vi "GV-MouseUP.vi"(7 "MouseLeave?":bool, 8 "error in (no error)":errorcluster, 9 "Coords":T1, 11 "Gviewer in":refnum<class "Gviewer.lvclass">) -> (0 "error out":errorcluster, 3 "Gviewer out":refnum<class "Gviewer.lvclass">)   [LabVIEW 2020, in "Sgraph_lib_V1.lvlib" / "Gviewer.lvclass"]
doc: "Andre Koelewijn, 24 jan 2021\n\nAction when in the Gviewer graph the mouse button is released"
uses:
  Gviewer.lvclass
  <vilib>/Utility/miscctls.llb/LVPoint32TypeDef.ctl
  Gviewer.lvclass/Gviewer.ctl
  <vilib>/Utility/cursorutil.llb/Set Cursor (Icon Pict).vi
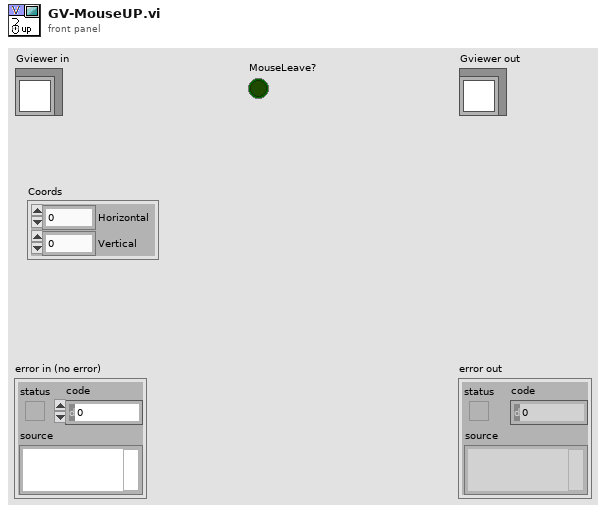
[diagram p1: front panel]
types:
  T1 = typedef "LVPoint32TypeDef.ctl" = cluster{"Horizontal":i32, "Vertical":i32}
  T2 = typedef "Sgraph_lib_V1.lvlib/Gviewer.lvclass/Typedef_Live.ctl" = enum16{"Live View", "Freeze"}
  T3 = typedef "LVPositionTypeDef.ctl" = cluster{"Left":i32, "Top":i32}
  T4 = typedef "LVBoundsTypeDef.ctl" = cluster{"Width":u32, "Height":u32}
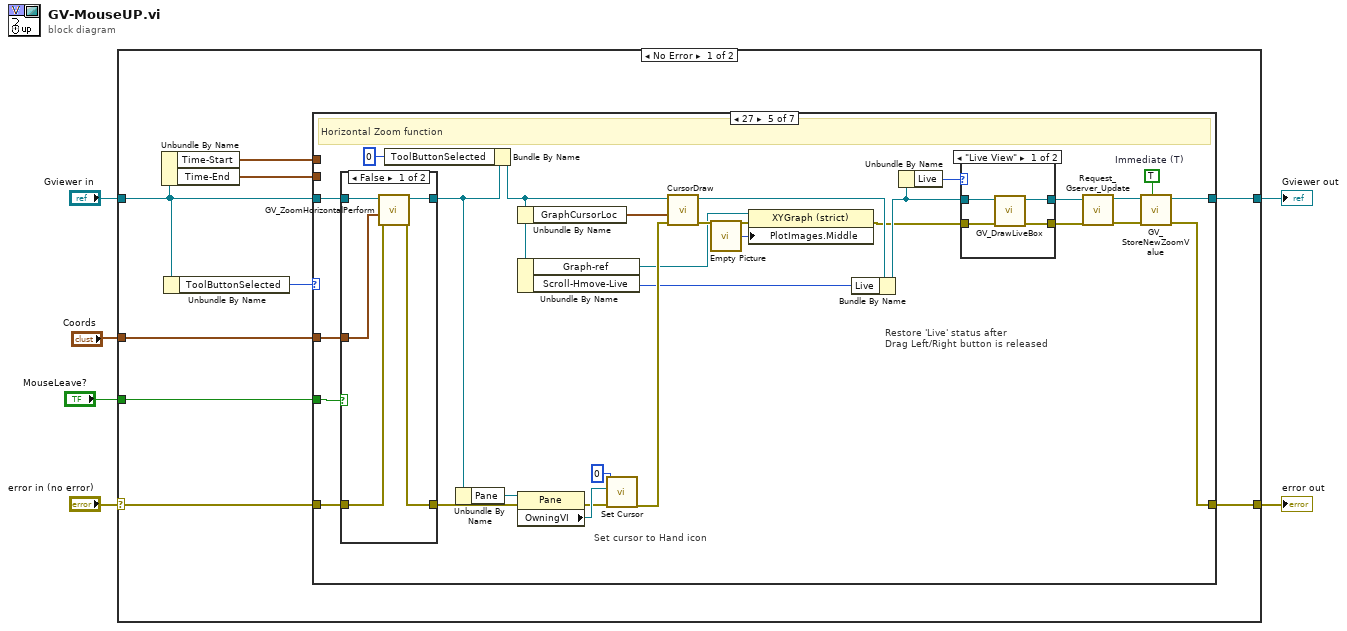
[diagram p0: block diagram]
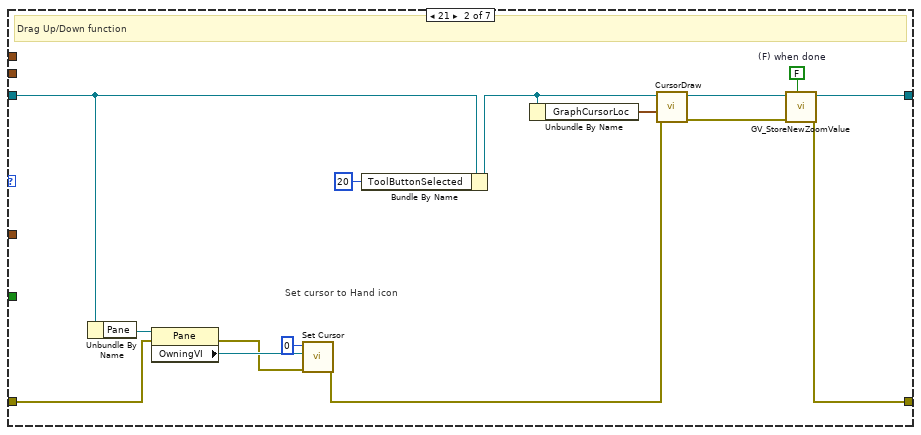
[diagram p3: hidden frame]
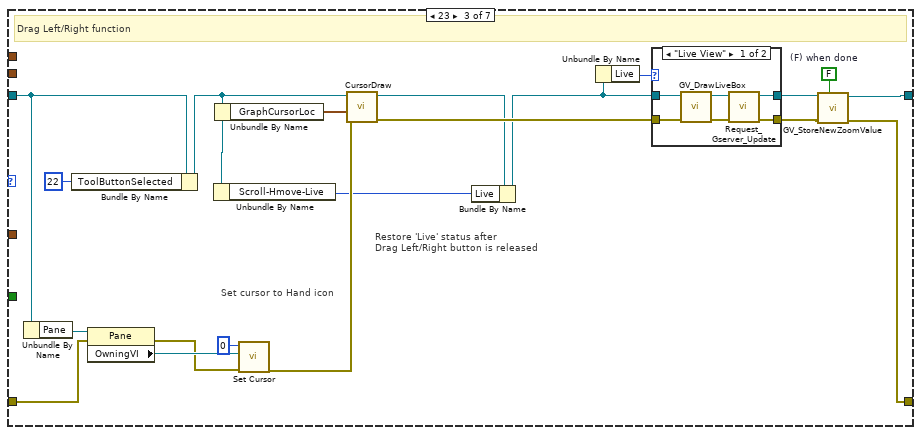
[diagram p4: hidden frame]
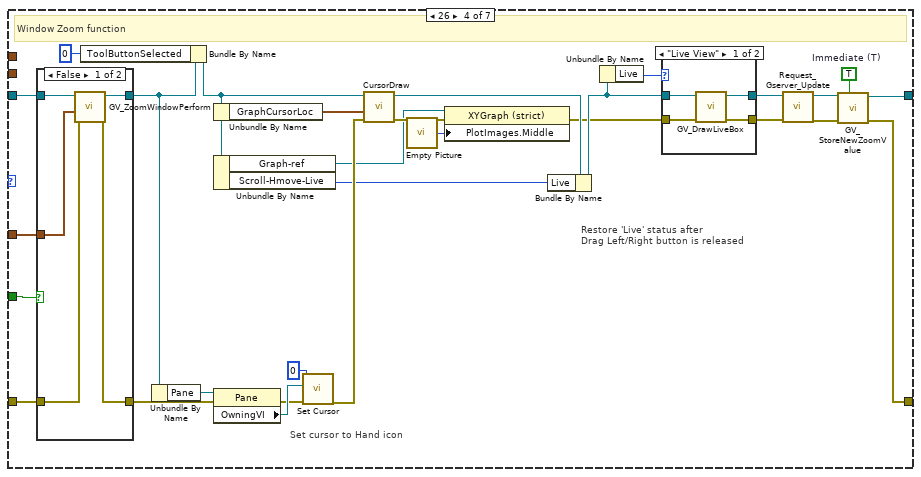
[diagram p6: hidden frame]
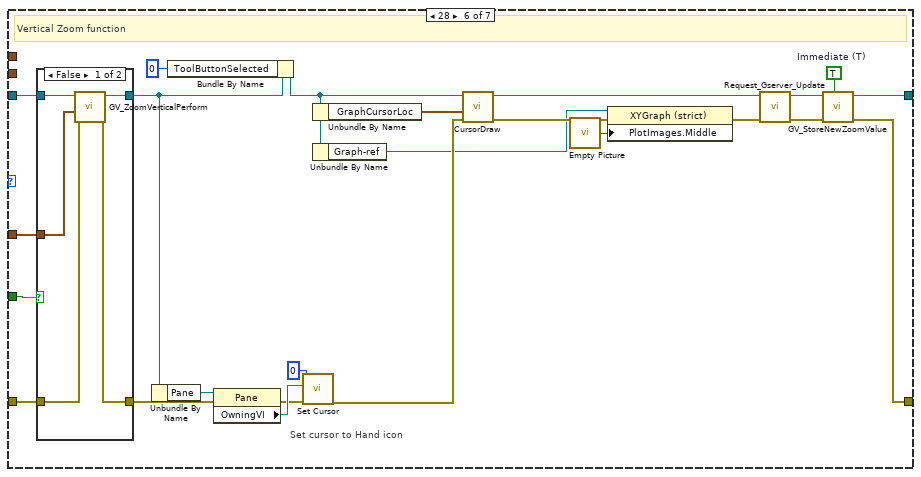
[diagram p11: hidden frame]
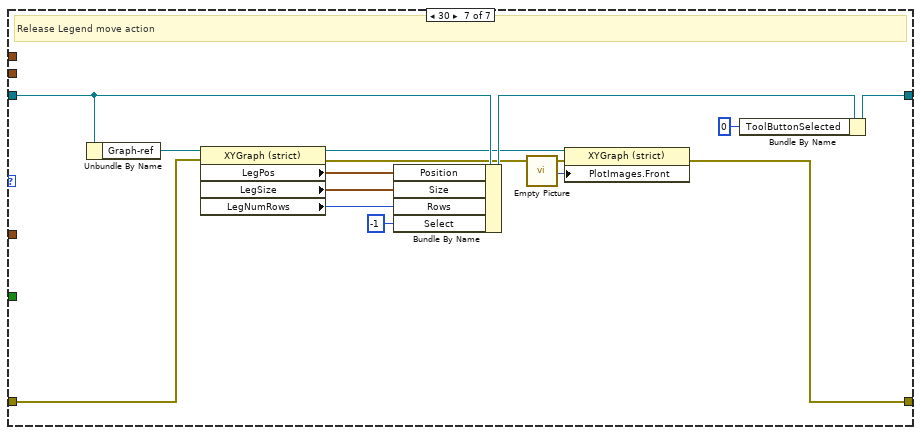
[diagram p13: hidden frame]
diagram:
  n1 = case shown="No Error" "error in (no error)" {
    selector: "error in (no error)" -> [w14 w191]
    tunnel: [w13 w191] -> w5
    tunnel: [w15 w190] -> w3
    tunnel: "Gviewer in" -> [w11 w190]
    tunnel: "Coords" -> [w8 _]
    tunnel: "MouseLeave?" -> [w7 _]
    frame No Error {
      n2 = Unbundle By Name(w11) -> ("Time-Start"=w10:timestamp, "Time-End"=w9:timestamp)
      n3 = Unbundle By Name(w11) -> ("ToolButtonSelected"=w12:i32)
      n4 = case shown="27" w12 {
        tunnel: w11 -> [w16 w30 w50 w73 w118 w157 w181]
        tunnel: w14 -> [w17 w26 w46 w71 w116 w155 w176]
        tunnel: [w17 w18 w33 w62 w104 w146 w177] -> w13
        tunnel: [w16 w20 w34 w61 w103 w148 w188] -> w15
        tunnel: w10 -> [_ _ _ _ _ _ _]
        tunnel: w9 -> [_ _ _ _ _ _ _]
        tunnel: w8 -> [_ _ _ w70 w115 w154 _]
        tunnel: w7 -> [_ _ _ w68 w113 w152 _]
        frame Default {
          # "other"
        }
        frame 21 {
          w22 = FALSE  # (F) when done
          # "Set cursor to Hand icon"
          # "Drag Up/Down function"
          n5 = Unbundle By Name(w30) -> ("Pane"=w29:refnum<vi>)
          n6 = property class="Pane"(reference=w29, error in=w26) -> (error out=w27:errorcluster, "OwningVI"=w28:refnum<vi>)  [unwired: 1 out]
          n7 = call-poly <vilib>:"Set Cursor.vi"("error in (no error)"=w27, "VI reference (current VI)"=w28, "icon"=u16 0) -> ("error out"=w23:errorcluster)  [unwired: 7 in, 1 out]
          n8 = Bundle By Name(cluster=w30, "ToolButtonSelected"=20) -> (w24:refnum<class "Gviewer.lvclass">)
          n9 = Unbundle By Name(w24) -> ("GraphCursorLoc"=w25:T1)
          n10 = call "CursorDraw.vi"("error in (no error)"=w23, "Coords"=w25, "Gviewer in"=w24) -> ("error out"=w19:errorcluster, "Gviewer out"=w21:refnum<class "Gviewer.lvclass">)  [unwired: 7 in]
          n11 = call "GV_StoreNewZoomValue.vi"("Immediate"=w22, "error in (no error)"=w19, "Gviewer in"=w21) -> ("error out"=w18:errorcluster, "Gviewer out"=w20:refnum<class "Gviewer.lvclass">)  [unwired: 7 in]
        }
        frame 23 {
          w37 = FALSE  # (F) when done
          # "Restore 'Live' status after\nDrag Left/Right button is released"
          # "Set cursor to Hand icon"
          # "Drag Left/Right function"
          n12 = Unbundle By Name(w50) -> ("Pane"=w49:refnum<vi>)
          n13 = Bundle By Name(cluster=w50, "ToolButtonSelected"=22) -> (w39:refnum<class "Gviewer.lvclass">)
          n14 = property class="Pane"(reference=w49, error in=w46) -> (error out=w47:errorcluster, "OwningVI"=w48:refnum<vi>)  [unwired: 1 out]
          n15 = Unbundle By Name(w39) -> ("Scroll-Hmove-Live"=w43:T2)
          n16 = Unbundle By Name(w39) -> ("GraphCursorLoc"=w45:T1)
          n17 = call-poly <vilib>:"Set Cursor.vi"("error in (no error)"=w47, "VI reference (current VI)"=w48, "icon"=u16 0) -> ("error out"=w44:errorcluster)  [unwired: 7 in, 1 out]
          n18 = call "CursorDraw.vi"("error in (no error)"=w44, "Coords"=w45, "Gviewer in"=w39) -> ("error out"=w41:errorcluster, "Gviewer out"=w38:refnum<class "Gviewer.lvclass">)  [unwired: 7 in]
          n19 = Bundle By Name(cluster=w38, "Live"=w43) -> (w40:refnum<class "Gviewer.lvclass">)
          n20 = Unbundle By Name(w40) -> ("Live"=w42:T2)
          n21 = case shown="\"Live View\"" w42 {
            tunnel: w40 -> [w58 w60]
            tunnel: [w54 w60] -> w35
            tunnel: w41 -> [w57 w59]
            tunnel: [w53 w59] -> w36
            frame "Live View" {
              n22 = call "GV_DrawLiveBox.vi"("error in (no error)"=w57, "Gviewer in"=w58) -> ("error out"=w55:errorcluster, "Gviewer out"=w56:refnum<class "Gviewer.lvclass">)  [unwired: 8 in]
              n23 = call "Request_Gserver_Update.vi"("error in (no error)"=w55, "Gviewer in"=w56) -> ("error out"=w53:errorcluster, "Gviewer out"=w54:refnum<class "Gviewer.lvclass">)  [unwired: 8 in]
            }
            frame "Freeze" {
            }
          }
          n24 = call "GV_StoreNewZoomValue.vi"("Immediate"=w37, "error in (no error)"=w36, "Gviewer in"=w35) -> ("error out"=w33:errorcluster, "Gviewer out"=w34:refnum<class "Gviewer.lvclass">)  [unwired: 7 in]
        }
        frame 26 {
          w65 = TRUE  # Immediate (T)
          # "Restore 'Live' status after\nDrag Left/Right button is released"
          # "Set cursor to Hand icon"
          # "Window Zoom function"
          n25 = case shown="False" w68 {
            tunnel: w73 -> [w94 w96]
            tunnel: [w93 w95] -> w72
            tunnel: w71 -> [w92 w95]
            tunnel: w70 -> [w91 _]
            tunnel: [w90 w96] -> w69
            frame False {
              n26 = call "GV_ZoomWindowPerform.vi"("error in (no error)"=w92, "Coords"=w91, "Gviewer in"=w94) -> ("error out"=w93:errorcluster, "Gviewer out"=w90:refnum<class "Gviewer.lvclass">)  [unwired: 7 in]
            }
            frame True {
            }
          }
          n27 = Bundle By Name(cluster=w69, "ToolButtonSelected"=0) -> (w79:refnum<class "Gviewer.lvclass">)
          n28 = Unbundle By Name(w69) -> ("Pane"=w87:refnum<vi>)
          n29 = Unbundle By Name(w79) -> ("GraphCursorLoc"=w84:T1)
          n30 = Unbundle By Name(w79) -> ("Graph-ref"=w74:refnum<vi>, "Scroll-Hmove-Live"=w82:T2)
          n31 = property class="Pane"(reference=w87, error in=w72) -> (error out=w85:errorcluster, "OwningVI"=w86:refnum<vi>)  [unwired: 1 out]
          n32 = call-poly <vilib>:"Set Cursor.vi"("error in (no error)"=w85, "VI reference (current VI)"=w86, "icon"=u16 0) -> ("error out"=w83:errorcluster)  [unwired: 7 in, 1 out]
          n33 = call "CursorDraw.vi"("error in (no error)"=w83, "Coords"=w84, "Gviewer in"=w79) -> ("error out"=w77:errorcluster, "Gviewer out"=w78:refnum<class "Gviewer.lvclass">)  [unwired: 7 in]
          n34 = call "Empty Picture"() -> ("empty picture"=w75:picture)
          n35 = property class="XYGraph (strict)"(reference=w74, error in=w77, "PlotImages.Middle"=w75) -> (error out=w76:errorcluster)  [unwired: 1 out]
          n36 = Bundle By Name(cluster=w78, "Live"=w82) -> (w80:refnum<class "Gviewer.lvclass">)
          n37 = Unbundle By Name(w80) -> ("Live"=w81:T2)
          n38 = case shown="\"Live View\"" w81 {
            tunnel: w80 -> [w100 w102]
            tunnel: [w98 w102] -> w67
            tunnel: w76 -> [w99 w101]
            tunnel: [w97 w101] -> w66
            frame "Live View" {
              n39 = call "GV_DrawLiveBox.vi"("error in (no error)"=w99, "Gviewer in"=w100) -> ("error out"=w97:errorcluster, "Gviewer out"=w98:refnum<class "Gviewer.lvclass">)  [unwired: 8 in]
            }
            frame "Freeze" {
            }
          }
          n40 = call "Request_Gserver_Update.vi"("error in (no error)"=w66, "Gviewer in"=w67) -> ("error out"=w64:errorcluster, "Gviewer out"=w63:refnum<class "Gviewer.lvclass">)  [unwired: 8 in]
          n41 = call "GV_StoreNewZoomValue.vi"("Immediate"=w65, "error in (no error)"=w64, "Gviewer in"=w63) -> ("error out"=w62:errorcluster, "Gviewer out"=w61:refnum<class "Gviewer.lvclass">)  [unwired: 7 in]
        }
        frame 27 {
          w107 = TRUE  # Immediate (T)
          # "Restore 'Live' status after\nDrag Left/Right button is released"
          # "Set cursor to Hand icon"
          # "Horizontal Zoom function"
          n42 = case shown="False" w113 {
            tunnel: w118 -> [w142 w144]
            tunnel: [w141 w143] -> w117
            tunnel: w116 -> [w140 w143]
            tunnel: w115 -> [w139 _]
            tunnel: [w138 w144] -> w114
            frame False {
              n43 = call "GV_ZoomHorizontalPerform.vi"("error in (no error)"=w140, "Coords"=w139, "Gviewer in"=w142) -> ("error out"=w141:errorcluster, "Gviewer out"=w138:refnum<class "Gviewer.lvclass">)  [unwired: 7 in]
            }
            frame True {
            }
          }
          n44 = Bundle By Name(cluster=w114, "ToolButtonSelected"=0) -> (w123:refnum<class "Gviewer.lvclass">)
          n45 = Unbundle By Name(w114) -> ("Pane"=w129:refnum<vi>)
          n46 = Unbundle By Name(w123) -> ("GraphCursorLoc"=w126:T1)
          n47 = Unbundle By Name(w123) -> ("Graph-ref"=w119:refnum<vi>, "Scroll-Hmove-Live"=w124:T2)
          n48 = property class="Pane"(reference=w129, error in=w117) -> (error out=w127:errorcluster, "OwningVI"=w128:refnum<vi>)  [unwired: 1 out]
          n49 = call-poly <vilib>:"Set Cursor.vi"("error in (no error)"=w127, "VI reference (current VI)"=w128, "icon"=u16 0) -> ("error out"=w125:errorcluster)  [unwired: 7 in, 1 out]
          n50 = call "CursorDraw.vi"("error in (no error)"=w125, "Coords"=w126, "Gviewer in"=w123) -> ("error out"=w121:errorcluster, "Gviewer out"=w122:refnum<class "Gviewer.lvclass">)  [unwired: 7 in]
          n51 = call "Empty Picture"() -> ("empty picture"=w120:picture)
          n52 = property class="XYGraph (strict)"(reference=w119, error in=w121, "PlotImages.Middle"=w120) -> (error out=w108:errorcluster)  [unwired: 1 out]
          n53 = Bundle By Name(cluster=w122, "Live"=w124) -> (w111:refnum<class "Gviewer.lvclass">)
          n54 = Unbundle By Name(w111) -> ("Live"=w112:T2)
          n55 = case shown="\"Live View\"" w112 {
            tunnel: w111 -> [w135 w137]
            tunnel: [w133 w137] -> w110
            tunnel: w108 -> [w134 w136]
            tunnel: [w132 w136] -> w109
            frame "Live View" {
              n56 = call "GV_DrawLiveBox.vi"("error in (no error)"=w134, "Gviewer in"=w135) -> ("error out"=w132:errorcluster, "Gviewer out"=w133:refnum<class "Gviewer.lvclass">)  [unwired: 8 in]
            }
            frame "Freeze" {
            }
          }
          n57 = call "Request_Gserver_Update.vi"("error in (no error)"=w109, "Gviewer in"=w110) -> ("error out"=w105:errorcluster, "Gviewer out"=w106:refnum<class "Gviewer.lvclass">)  [unwired: 8 in]
          n58 = call "GV_StoreNewZoomValue.vi"("Immediate"=w107, "error in (no error)"=w105, "Gviewer in"=w106) -> ("error out"=w104:errorcluster, "Gviewer out"=w103:refnum<class "Gviewer.lvclass">)  [unwired: 7 in]
        }
        frame 28 {
          w145 = TRUE  # Immediate (T)
          # "Set cursor to Hand icon"
          # "Vertical Zoom function"
          n59 = case shown="False" w152 {
            tunnel: w157 -> [w173 w175]
            tunnel: [w172 w174] -> w156
            tunnel: w155 -> [w171 w174]
            tunnel: w154 -> [w170 _]
            tunnel: [w169 w175] -> w153
            frame False {
              n60 = call "GV_ZoomVerticalPerform.vi"("error in (no error)"=w171, "Coords"=w170, "Gviewer in"=w173) -> ("error out"=w172:errorcluster, "Gviewer out"=w169:refnum<class "Gviewer.lvclass">)  [unwired: 7 in]
            }
            frame True {
            }
          }
          n61 = Unbundle By Name(w153) -> ("Pane"=w166:refnum<vi>)
          n62 = Bundle By Name(cluster=w153, "ToolButtonSelected"=0) -> (w161:refnum<class "Gviewer.lvclass">)
          n63 = property class="Pane"(reference=w166, error in=w156) -> (error out=w164:errorcluster, "OwningVI"=w165:refnum<vi>)  [unwired: 1 out]
          n64 = call-poly <vilib>:"Set Cursor.vi"("error in (no error)"=w164, "VI reference (current VI)"=w165, "icon"=u16 0) -> ("error out"=w162:errorcluster)  [unwired: 7 in, 1 out]
          n65 = Unbundle By Name(w161) -> ("GraphCursorLoc"=w163:T1)
          n66 = Unbundle By Name(w161) -> ("Graph-ref"=w158:refnum<vi>)
          n67 = call "CursorDraw.vi"("error in (no error)"=w162, "Coords"=w163, "Gviewer in"=w161) -> ("error out"=w160:errorcluster, "Gviewer out"=w150:refnum<class "Gviewer.lvclass">)  [unwired: 7 in]
          n68 = call "Empty Picture"() -> ("empty picture"=w159:picture)
          n69 = property class="XYGraph (strict)"(reference=w158, error in=w160, "PlotImages.Middle"=w159) -> (error out=w151:errorcluster)  [unwired: 1 out]
          n70 = call "Request_Gserver_Update.vi"("error in (no error)"=w151, "Gviewer in"=w150) -> ("error out"=w147:errorcluster, "Gviewer out"=w149:refnum<class "Gviewer.lvclass">)  [unwired: 8 in]
          n71 = call "GV_StoreNewZoomValue.vi"("Immediate"=w145, "error in (no error)"=w147, "Gviewer in"=w149) -> ("error out"=w146:errorcluster, "Gviewer out"=w148:refnum<class "Gviewer.lvclass">)  [unwired: 7 in]
        }
        frame 30 {
          # "Release Legend move action"
          n72 = Unbundle By Name(w181) -> ("Graph-ref"=w186:refnum<vi>)
          n73 = property class="XYGraph (strict)"(reference=w186, error in=w176) -> (reference out=w180:refnum<vi>, error out=w178:errorcluster, "LegPos"=w185:T3, "LegSize"=w184:T4, "LegNumRows"=w183:u32)
          n74 = Bundle By Name(cluster=w181, "Position"=w185, "Size"=w184, "Rows"=w183, "Select"=-1 ("Legend.Select")) -> (w182:refnum<class "Gviewer.lvclass">)
          n75 = call "Empty Picture"() -> ("empty picture"=w179:picture)
          n76 = property class="XYGraph (strict)"(reference=w180, error in=w178, "PlotImages.Front"=w179) -> (error out=w177:errorcluster)  [unwired: 1 out]
          n77 = Bundle By Name(cluster=w182, "ToolButtonSelected"=0) -> (w188:refnum<class "Gviewer.lvclass">)
        }
      }
    }
    frame Error {
    }
  }
  "error out" <- w5
  "Gviewer out" <- w3
